vi "LPFilt.vi"(1 "LP%":dbl=0.01, 2 "Input":dbl) -> (0 "Filtered":dbl)   [LabVIEW 2013]
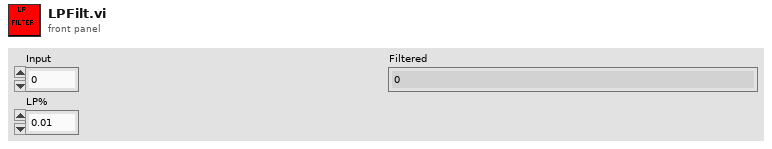
[diagram p1: front panel]
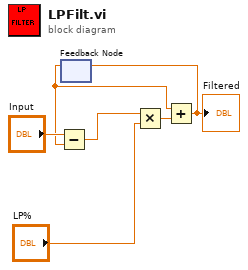
[diagram p0: block diagram]
diagram:
  n1 = feedback #1() -> (w4:dbl)  [unwired: 1 in]
  n2 = Subtract(x="Input", y=w4) -> (x-y=w6:dbl)
  n3 = Multiply(x=w6, y="LP%") -> (x*y=w3:dbl)
  n4 = Add(x=w4, y=w3) -> (x+y=w2:dbl)
  "Filtered" <- w2
  n5 = feedback-in #1(w2) -> ()
